vi "OpenG Search 1D Array Template.vi"(0 "Array":i32[](array[numeric]), 2 "Element Data":i32, 3 "Start Index (0)":i32) -> (7 "Indices of Elements":i32[](array[numeric]))   [LabVIEW 2018]
doc: "Searches for all element data matches in array"
panel:
  # "[OpenG VI Tags] ***Do Not Remove***\n\nSVN Revision = 990\nSVN Revision Date = 2009-07-18 07:14:13 -0700 (Sat, 18 Jul 2009)\nPackage = oglib_array-3.0.0-1\nDepends ="
  # "Search 1D Array.vi\n\nSearches for all element data matches in array\n\nPlease visit http://www.OpenG.org to learn about the\nOpen Source LabVIEW software movement.\n\nNOTICE -- YOU MUST LEAVE THIS NOTICE IN PLACE.  PER THE TERMS OF THE LICENSE BELOW, YOU MAY SUBLICENSE THIS SOFTWARE \nIN ANY WAY THAT DOES NOT CONFLICT WITH THIS LICENSE.\n\n### BSD License (http://www.opensource.org/licenses/bsd-license.php) Begin ###\n \nCopyright (c) 2005, MKS Instruments, Inc., author: Doug Femec<doug_femec@mksinst.com>, IM dafemec\n\nAll rights reserved.\n\nRedistribution and use in source and binary forms, with or without modification, are permitted provided that the following conditions are met:\n\n    * Redistributions of source code must retain the above copyright notice, this list of conditions and the following disclaimer.\n    * Redistributions in binary form must reproduce the above copyright notice, this list of conditions and the following disclaimer in the \n       documentation and/or other materials provided with the distribution.\n    * Neither the name of SciWare, James Kring, Inc., nor the names of its contributors may be used to endorse or promote products derived \n       from this software without specific prior written permission.\n\nTHIS SOFTWARE IS PROVIDED BY THE COPYRIGHT HOLDERS AND CONTRIBUTORS \"AS IS\" AND ANY EXPRESS OR IMPLIED WARRANTIES, \nINCLUDING, BUT NOT LIMITED TO, THE IMPLIED WARRANTIES OF MERCHANTABILITY AND FITNESS FOR A PARTICULAR PURPOSE ARE \nDISCLAIMED. IN NO EVENT SHALL THE COPYRIGHT OWNER OR CONTRIBUTORS BE LIABLE FOR ANY DIRECT, INDIRECT, INCIDENTAL,\n SPECIAL, EXEMPLARY, OR CONSEQUENTIAL DAMAGES (INCLUDING, BUT NOT LIMITED TO, PROCUREMENT OF SUBSTITUTE GOODS OR \nSERVICES; LOSS OF USE, DATA, OR PROFITS; OR BUSINESS INTERRUPTION) HOWEVER CAUSED AND ON ANY THEORY OF LIABILITY, \nWHETHER IN CONTRACT, STRICT LIABILITY, OR TORT (INCLUDING NEGLIGENCE OR OTHERWISE) ARISING IN ANY WAY OUT OF THE USE \nOF THIS SOFTWARE, EVEN IF ADVISED OF THE POSSIBILITY OF SUCH DAMAGE.\n\n### BSD License End ###"
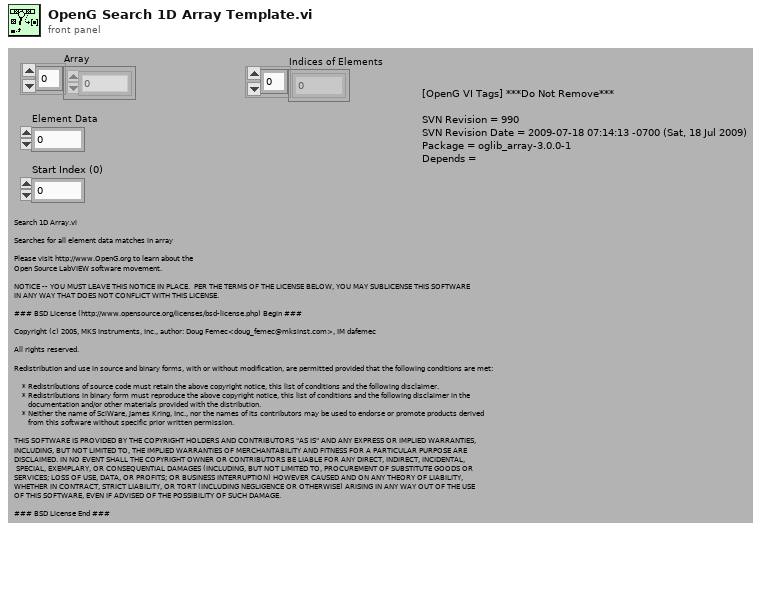
[diagram p1: front panel]
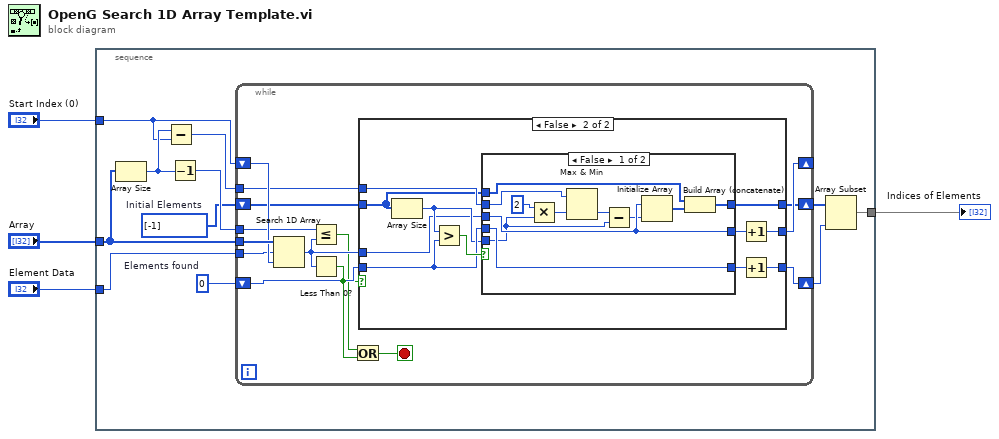
[diagram p0: block diagram]
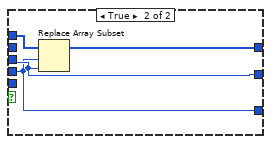
[diagram p3: hidden frame]
diagram:
  n1 = stacked-sequence {
    tunnel: [w7] -> w4
    tunnel: "Array" -> [w5]
    tunnel: "Start Index (0)" -> [w8]
    tunnel: "Element Data" -> [w6]
    frame #0 {
      w9 = i32[] [-1]  # Initial Elements
      w11 = 0  # Elements found
      n2 = Array Size(array=w5) -> (size(s)=w10:i32)
      n3 = Subtract(x=w10, y=w8) -> (x-y=w14:i32)
      n4 = Decrement(x=w10) -> (x-1=w15:i32)
      n5 = while {
        tunnel: w5 -> [w29]
        shift-right: [w26] -> _
        shift-left: w8 -> [w28]
        shift-right: [w22] -> w12
        shift-left: w9 -> [w25]
        shift-right: [w23] -> w13
        shift-left: w11 -> [w24]
        tunnel: w6 -> [w27]
        tunnel: w14 -> [w21]
        tunnel: w15 -> [w20]
        stop <- w16 stop-if-true
        n6 = Search 1D Array(1D array=w29, element=w27, start index (0)=w28) -> (index of element=w19:i32)
        n7 = Less Or Equal?(x=w20, y=w19) -> (x <= y?=w18:bool)
        n8 = Less Than 0?(x=w19) -> (x < 0?=w17:bool)
        n9 = Or(x=w18, y=w17) -> (x .or. y?=w16:bool)
        n10 = case shown="False" w17 {
          tunnel: [w30 w39] -> w26
          tunnel: w25 -> [w32 w34]
          tunnel: w24 -> [w31 w42]
          tunnel: [w31 w35] -> w23
          tunnel: [w32 w41] -> w22
          tunnel: w21 -> [_ w38]
          tunnel: w19 -> [w30 w33]
          frame True {
          }
          frame False {
            n11 = Array Size(array=w34) -> (size(s)=w37:i32)
            n12 = Greater?(x=w37, y=w42) -> (0:w43:bool)
            n13 = case shown="False" w43 {
              tunnel: w34 -> [w53 w58]
              tunnel: w42 -> [w50 w55]
              tunnel: [w52 w57] -> w41
              tunnel: w33 -> [w54 w56]
              tunnel: [w54 w56] -> w40
              tunnel: w38 -> [w47 _]
              tunnel: w37 -> [w45 _]
              tunnel: [w50 w55] -> w36
              frame False {
                n14 = Multiply(x=2 ("y"), y=w45) -> (x*y=w48:i32)
                n15 = Max & Min(x=w47, y=w48) -> (min(x,y)=w46:i32)  [unwired: 1 out]
                n16 = Subtract(x=w46, y=w45) -> (x-y=w44:i32)
                n17 = Initialize Array(w54, w44) -> (w51:i32[])
                n18 = Build Array (concatenate)(w53, w51) -> (w52:i32[])
              }
              frame True {
                n19 = Replace Array Subset(array=w58, new element=w56, index=w55) -> (w57:i32[])
              }
            }
            n20 = Increment(x=w40) -> (x+1=w39:i32)
            n21 = Increment(x=w36) -> (x+1=w35:i32)
          }
        }
      }
      n22 = Array Subset(array=w12, length=w13) -> (w7:i32[])  [unwired: 1 in]
    }
  }
  "Indices of Elements" <- w4
